vi "Init.vi"(8 "error in (no error)":errorcluster, 9 "Value":refnum<vi>, 10 "State":refnum<vi>) -> (0 "error out":errorcluster, 3 "Simple TCP Handler out":refnum<class "Simple TCP Handler.lvclass">)   [LabVIEW 2020, in "VectoScratch.lvlib" / "Simple TCP Handler.lvclass"]
uses:
  Simple TCP Handler.lvclass
  Vecto/Connection State.ctl
  Simple TCP Handler.lvclass/Simple TCP Handler.ctl
  Vecto/Vecto.lvlib
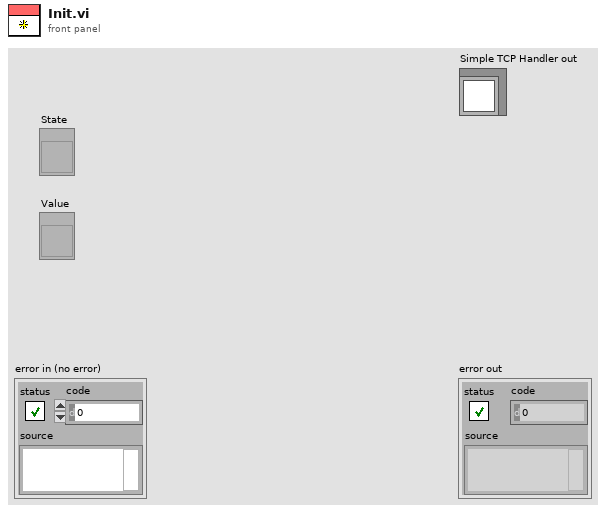
[diagram p1: front panel]
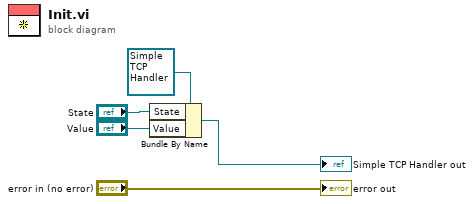
[diagram p0: block diagram]
diagram:
  n1 = Bundle By Name(cluster=refnum<class "Simple TCP Handler.lvclass"> refnum ("Simple TCP Handler in"), "State"="State", "Value"="Value") -> (→"Simple TCP Handler out":refnum<class "Simple TCP Handler.lvclass">)
  "error out" <- "error in (no error)"
